vi "AnyBuilderBeginRepeatedNestedMessageElement.vi"(8 "error in":errorcluster, 11 "gRPCid in":T1) -> (0 "error out":errorcluster, 2 "Nested Element ID":T1, 3 "gRPCid out":T1)   [LabVIEW 2019, in "grpc-lvsupport.lvlib"]
uses:
  grpc-lvsupport.lvlib
  Shared/grpcId.ctl
  <vilib>/Utility/error.llb/Error Cluster From Error Code.vi
  <resource>/labview_grpc_server.dll
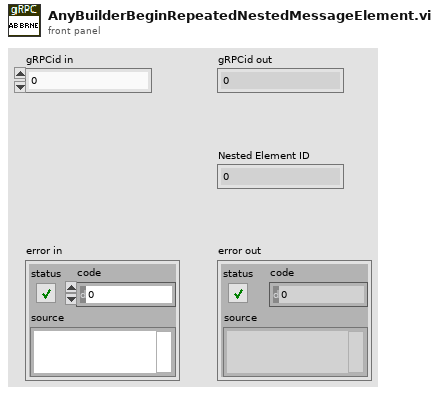
[diagram p1: front panel]
types:
  T1 = typedef "grpc-lvsupport.lvlib/grpcId.ctl" = u64
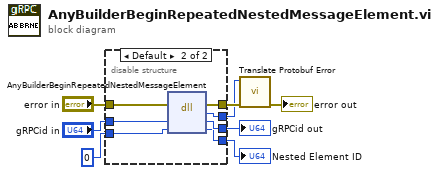
[diagram p0: block diagram]
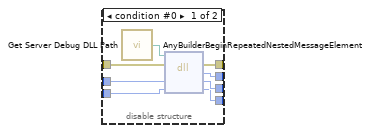
[diagram p2: hidden frame]
diagram:
  n1 = disable-structure shown="Default" {
    disable-tunnel: "error in" -> [w16 w23]
    disable-tunnel: [w15 w22] -> w7
    disable-tunnel: "gRPCid in" -> [w14 w21]
    disable-tunnel: [w13 w20] -> w5
    disable-tunnel: [w11 w19] -> w4
    disable-tunnel: [w10 w18] -> w2
    disable-tunnel: u64 0 ("nestedId") -> [w9 w17]
    frame condition #0 {
      n2 = call "Get Server Debug DLL Path.vi"() -> ("DLL Path"=w12:path)
      n3 = dll-call lib="?" fn="AnyBuilderBeginRepeatedNestedMessageElement"(path in=w12, error in=w16, "builderId"=w14, "nestedId"=w9) -> (error out=w15:errorcluster, "return type"=w10:i32, "builderId"=w13:u64, "nestedId"=w11:u64)  [unwired: 1 in, 1 out]
    }
    frame condition #1 (active) {
      n4 = dll-call lib="C:/Program Files (x86)/National Instruments/LabVIEW 2024/resource/labview_grpc_server.*" fn="AnyBuilderBeginRepeatedNestedMessageElement"(error in=w23, "builderId"=w21, "nestedId"=w17) -> (error out=w22:errorcluster, "return type"=w18:i32, "builderId"=w20:u64, "nestedId"=w19:u64)  [unwired: 2 in, 1 out]
    }
  }
  "gRPCid out" <- w5
  "Nested Element ID" <- w4
  n5 = call "Translate Protobuf Error.vi"("error in"=w7, "Error Code"=w2) -> ("error out"=→"error out":errorcluster)  [unwired: 9 in]
